vi "Set Inkscape Ratio.vi"(1 "Image Size In":cluster{"Width":dbl, "Height":dbl}) -> (0 "Image Size Out":cluster{"Width":dbl, "Height":dbl})   [LabVIEW 2016]
uses:
  Global Variables.vi
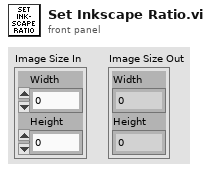
[diagram p1: front panel]
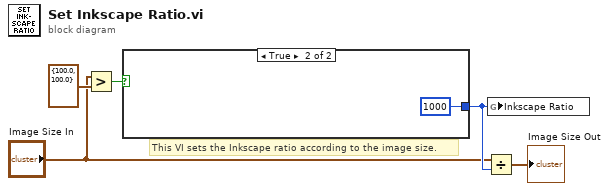
[diagram p0: block diagram]
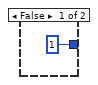
[diagram p2: hidden frame]
diagram:
  # "This VI sets the Inkscape ratio according to the image size."
  n1 = Greater?(x="Image Size In", y=cluster{"Width":dbl, "Height":dbl} {"Width"=100.0, "Height"=100.0}) -> (0:w4:bool)
  n2 = case shown="True" w4 {
    tunnel: [1 1000] -> w3
    frame False {
    }
    frame True {
    }
  }
  n3 = Divide(x="Image Size In", y=w3) -> (x/y=→"Image Size Out":cluster{"Width":dbl, "Height":dbl})
  n4 = global write "Global Variables.vi" "Inkscape Ratio"(w3) -> ()
